vi "Write reg.vi"(5 "Write type":enum16{"Normal", "Extended", "Extended Cycle"}(ring), 7 "Write USID":u8=7, 8 "error in (no error)":errorcluster, 9 "Write Data":u32[](array[numeric])=[128] format="%x", 10 "Write Address":u32, 11 "niDigital in":refnum<class "niDigital.lvclass">) -> (0 "error out":errorcluster, 3 "niDigital out":refnum<class "niDigital.lvclass">)   [LabVIEW 2020, in "niDigital.lvclass"]
uses:
  niDigital.lvclass
  <instrlib>/niDigital/niDigital.llb/niDigital Data Mapping.ctl
  <instrlib>/niDigital/niDigital.llb/niDigital Bit Order.ctl
  <instrlib>/niDigital/niDigital.llb/niDigital Selected Function.ctl
  <instrlib>/niDigital/niDigital.llb/niDigital Create Source Waveform (Serial).vi
  <instrlib>/niDigital/niDigital.llb/niDigital Write Source Waveform (Broadcast U32).vi
  <instrlib>/niDigital/niDigital.llb/niDigital Burst Pattern (Burst Only).vi
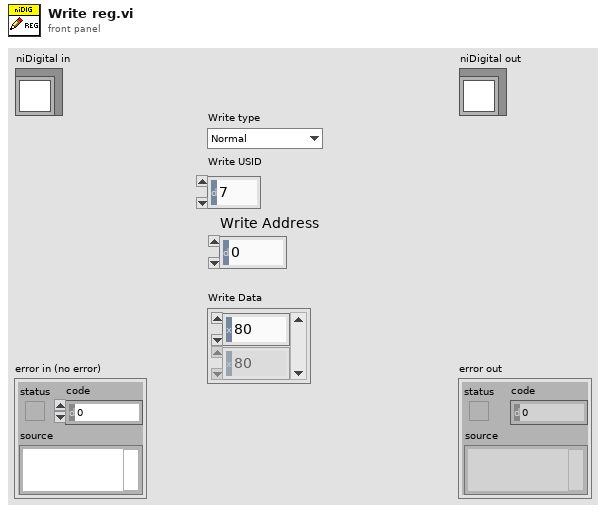
[diagram p1: front panel]
types:
  T1 = typedef "niDigital Selected Function.ctl" = i32
  T2 = typedef "niDigital Bit Order.ctl" = i32
  T3 = typedef "niDigital Data Mapping.ctl" = i32
  T4 = cluster{"Write Reg Pattern":string, "Ext Write Reg Pattern":string, "Cyc Ext Write Reg Pattern":string, "Read Reg Pattern":string}
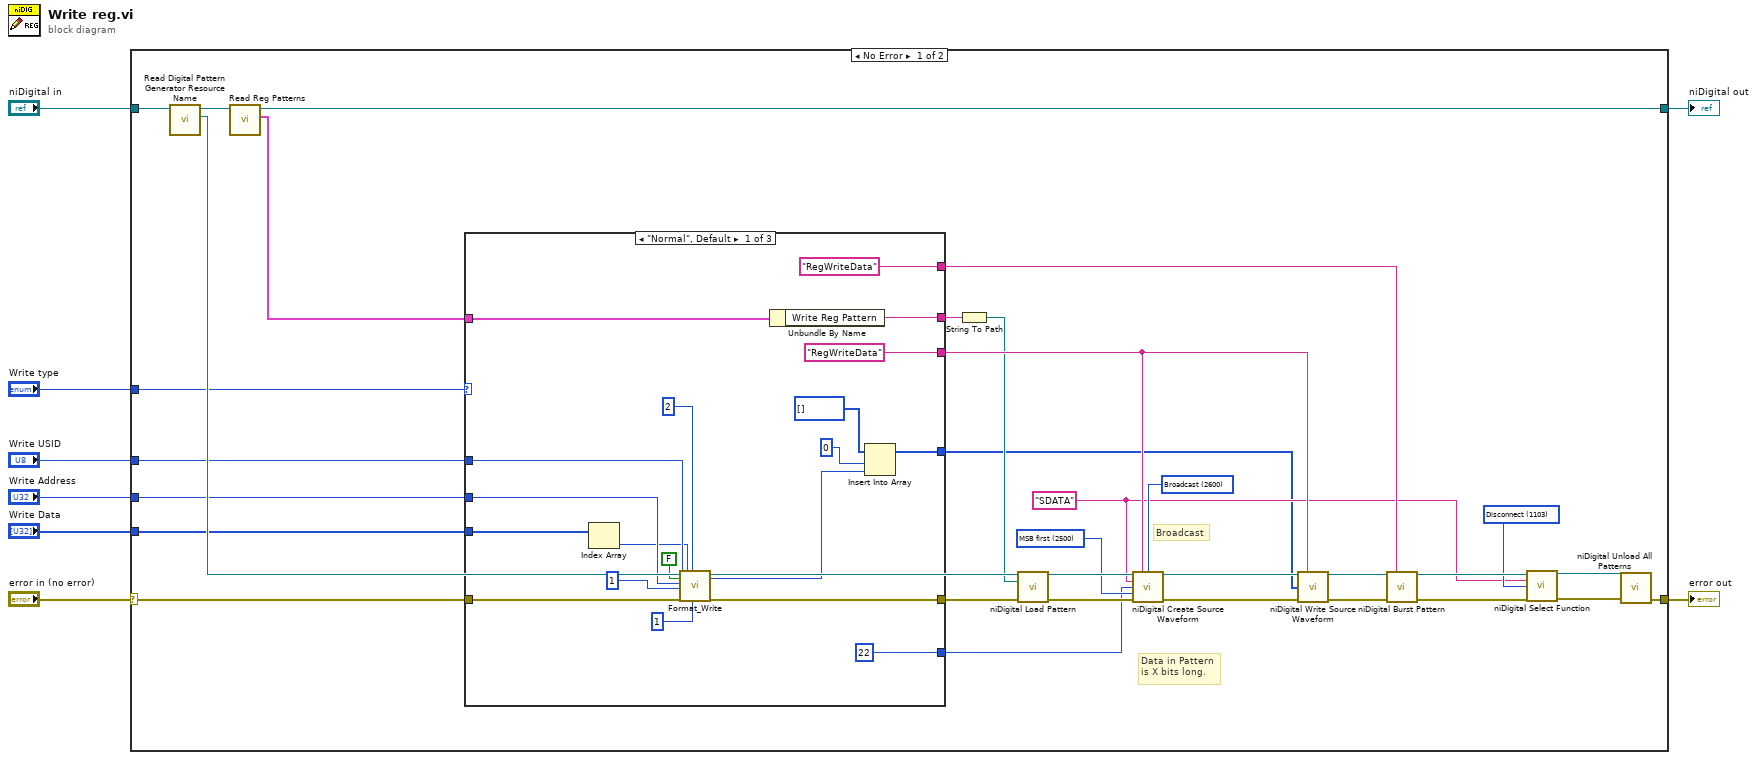
[diagram p0: block diagram]
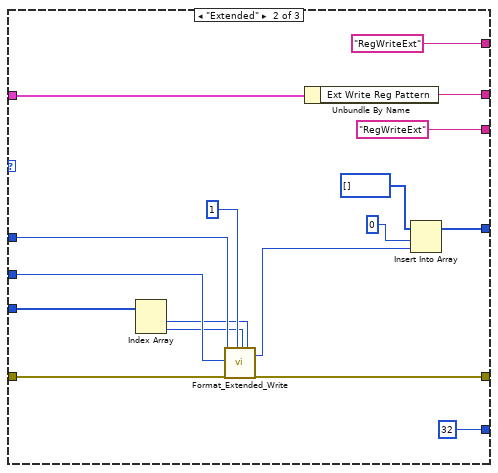
[diagram p2: hidden frame]
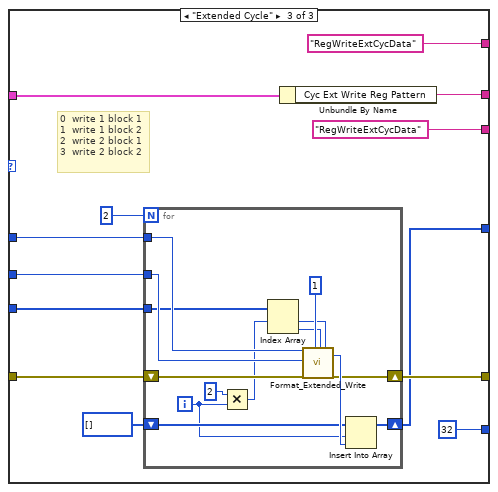
[diagram p3: hidden frame]
diagram:
  n1 = case shown="No Error" "error in (no error)" {
    selector: "error in (no error)" -> [w15 w105]
    tunnel: [w22 w105] -> w7
    tunnel: [w12 w104] -> w5
    tunnel: "niDigital in" -> [w24 w104]
    tunnel: "Write USID" -> [w17 _]
    tunnel: "Write Address" -> [w16 _]
    tunnel: "Write Data" -> [w9 _]
    tunnel: "Write type" -> [w10 _]
    frame No Error {
      w26 = T1 1103 items=["Digital"=1100, "PPMU"=1101, "Off"=1102, "Disconnect"=1103] ("function")
      w34 = T2 2500 items=["MSB first"=2500, "LSB first"=2501] ("bit order")
      w25 = "SDATA" ("Serial Channel List")
      w35 = T3 2600 items=["Broadcast"=2600, "Site Unique"=2601] ("data mapping")
      # "Data in Pattern\nis X bits long."
      # "Broadcast"
      n2 = call-dynamic "Read Digital Pattern Generator Resource Name.vi"("niDigital in"=w24) -> ("Digital Pattern Generator Resource Name"=w23:refnum<k15>, "niDigital out"=w13:refnum<class "niDigital.lvclass">)  [unwired: 9 in]
      n3 = call-dynamic "Read Reg Patterns.vi"("niDigital in"=w13) -> ("Reg Patterns"=w21:T4, "niDigital out"=w12:refnum<class "niDigital.lvclass">)  [unwired: 9 in]
      n4 = case shown="\"Normal\", Default" w10 {
        tunnel: ["RegWriteData" ("Write Reg source_start opcode") "RegWriteExt" ("Write Reg source_start opcode") "RegWriteExtCycData" ("Write Reg source_start opcode")] -> w33
        tunnel: ["RegWriteData" ("Write_Reg Pattern Name") "RegWriteExt" ("Write_Reg Pattern Name") "RegWriteExtCycData" ("Write_Reg Pattern Name")] -> w32
        tunnel: w21 -> [w57 w74 w87]
        tunnel: [w56 w73 w86] -> w20
        tunnel: [u32 22 ("y") u32 32 ("y") u32 32 ("y")] -> w18
        tunnel: w17 -> [w54 w66 w77]
        tunnel: w16 -> [w52 w67 w78]
        tunnel: w9 -> [w49 w70 w79]
        tunnel: w15 -> [w47 w69 w84]
        tunnel: [w46 w68 w83] -> w14
        tunnel: [w41 w60 w82] -> w11
        frame "Normal", Default {
          n5 = Index Array(array=w49) -> (element=w48:u32)  [unwired: 1 in]
          n6 = call "Format_Write.vi"("Source Address"=w54, "Register 0 Write?"=FALSE, "Address"=w52, "Address Parity"=u32 1, "error in (no error)"=w47, "Data"=w48, "CMD"=u32 2, "Data Parity"=u32 1) -> ("RFFE Write Word"=w42:u32, "error out"=w46:errorcluster)  [unwired: 10 in]
          n7 = Unbundle By Name(w57) -> ("Write Reg Pattern"=w56:string)
          n8 = Insert Into Array(array=u32[] [], index=0, new element=w42) -> (w41:u32[])
        }
        frame "Extended" {
          n9 = Index Array(array=w70) -> (element #1=w65:u32, element #2=w64:u32)  [unwired: 2 in]
          n10 = call "Format_Extended_Write.vi"("Source Address"=w66, "Address"=w67, "error in (no error)"=w69, "BC"=u32 1, "Data_Blk_2"=w64, "Data_Blk_1"=w65) -> ("RFFE Write Word"=w61:u32, "error out"=w68:errorcluster)  [unwired: 12 in]
          n11 = Unbundle By Name(w74) -> ("Ext Write Reg Pattern"=w73:string)
          n12 = Insert Into Array(array=u32[] [], index=0, new element=w61) -> (w60:u32[])
        }
        frame "Extended Cycle" {
          # "0  write 1 block 1\n1  write 1 block 2\n2  write 2 block 1\n3  write 2 block 2"
          n13 = for {
            N: 2 -> [_]
            shift-right: [w101] -> w82
            shift-left: u32[] [] -> [w102]
            tunnel: w77 -> [w99]
            tunnel: w78 -> [w98]
            shift-right: [w97] -> w83
            shift-left: w84 -> [w96]
            tunnel: w79 -> [w95]
            i -> [w94]
            n14 = Multiply(x=2, y=w94) -> (x*y=w92:i32)
            n15 = Index Array(array=w95, index #1=w92) -> (element #1=w91:u32, element #2=w90:u32)  [unwired: 1 in]
            n16 = call "Format_Extended_Write.vi"("Source Address"=w99, "Address"=w98, "error in (no error)"=w96, "BC"=u32 1, "Data_Blk_2"=w90, "Data_Blk_1"=w91) -> ("RFFE Write Word"=w103:u32, "error out"=w97:errorcluster)  [unwired: 12 in]
            n17 = Insert Into Array(array=w102, index=w94, new element=w103) -> (w101:u32[])
          }
          n18 = Unbundle By Name(w87) -> ("Cyc Ext Write Reg Pattern"=w86:string)
        }
      }
      n19 = String To Path(string=w20) -> (path=w19:path)
      n20 = call <instrlib>:"niDigital Load Pattern.vi"("instrument handle"=w23, "pattern file"=w19, "error in"=w14) -> ("instrument handle out"=w40:refnum<k15>, "error out"=w31:errorcluster)  [unwired: 11 in]
      n21 = call-poly <instrlib>:"niDigital Create Source Waveform.vi"("instrument handle"=w40, "waveform name"=w33, "data mapping"=w35, "pin list"=w25, "sample width"=w18, "bit order"=w34, "error in"=w31) -> ("instrument handle out"=w39:refnum<k15>, "error out"=w38:errorcluster)  [unwired: 7 in]
      n22 = call-poly <instrlib>:"niDigital Write Source Waveform.vi"("instrument handle"=w39, "waveform name"=w33, "waveform data"=w11, "error in"=w38) -> ("instrument handle out"=w36:refnum<k15>, "error out"=w37:errorcluster)  [unwired: 10 in]
      n23 = call-poly <instrlib>:"niDigital Burst Pattern.vi"("instrument handle"=w36, "start label"=w32, "error in"=w37) -> ("instrument handle out"=w30:refnum<k15>, "error out"=w28:errorcluster)  [unwired: 11 in]
      n24 = call <instrlib>:"niDigital Select Function.vi"("instrument handle"=w30, "channel list"=w25, "function"=w26, "error in"=w28) -> ("instrument handle out"=w29:refnum<k15>, "error out"=w27:errorcluster)  [unwired: 10 in]
      n25 = call <instrlib>:"niDigital Unload All Patterns.vi"("instrument handle"=w29, "error in"=w27) -> ("error out"=w22:errorcluster)  [unwired: 12 in, 1 out]
    }
    frame Error {
    }
  }
  "error out" <- w7
  "niDigital out" <- w5
